vi "Delete DUT.vi"(8 "error in (no error)":errorcluster, 10 "DUT (\"DUT1\")":string="DUT1", 11 "VISA resource name":refnum<visa-resource-name>) -> (0 "error out":errorcluster, 3 "VISA resource name out":refnum<visa-resource-name>)   [LabVIEW 2020, in "Rohde&Schwarz CMXP Base.lvlib"]
doc: "Deletes the DUT with the specified name.\n\nAttribute:\nRSCMXPBASE_ATTR_DUT_DELETE\n\nRemote-control command:\nDELete:DUT"
uses:
  <instrlib>/Rohde&Schwarz CMXP Base/Rohde&Schwarz CMXP Base.lvlib
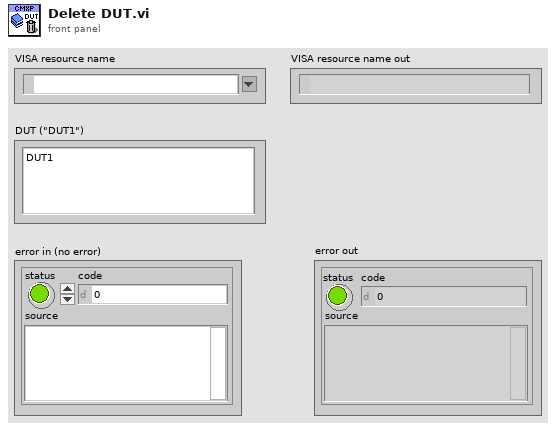
[diagram p1: front panel]
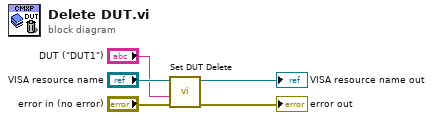
[diagram p0: block diagram]
diagram:
  n1 = call "Set DUT Delete"("error in (no error)"="error in (no error)", "DUT Delete ()"="DUT (\"DUT1\")", "instrument handle"="VISA resource name") -> ("error out"=→"error out":errorcluster, "instrument handle out"=→"VISA resource name out":refnum<visa-resource-name>)  [unwired: 7 in]
